vi "forloopStructureExample1.vi"() -> ()   [LabVIEW 2014]
panel:
  out "Even Numbers Array\nOutput Indicator":i32[](array[numeric])
  in  "Number of Iterations\nInput Control":i32
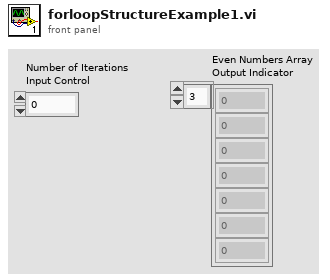
[diagram p1: front panel]
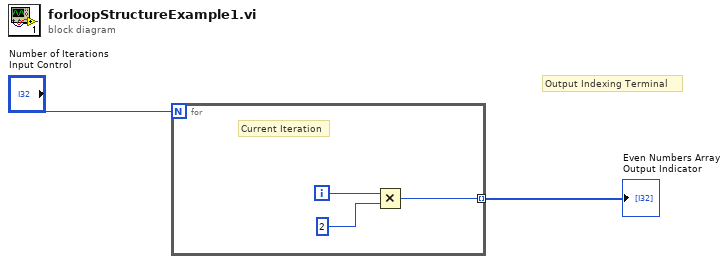
[diagram p0: block diagram]
diagram:
  # "Output Indexing Terminal"
  n1 = for {
    N: "Number of Iterations\nInput Control" -> [_]
    tunnel: [w3] -> w1 mode=indexing
    i -> [w5]
    # "Current Iteration"
    n2 = Multiply(x=w5, y=2) -> (x*y=w3:i32)
  }
  "Even Numbers Array\nOutput Indicator" <- w1
